vi "serialize.ob.cmd.vi"(11 "OrderBook.Commands.in":T1[](array[typedef])=[{"type"=enum."AddOrder", "side"=66, "orderId "=48, "quantity"=20000, "symbol"=4702127773838221344, "price"=9050, "executed.qty"=0, "canceled.qty"=0, "remaining.qty"=0, "seconds"=0, "nanoseconds"=0, "Add"=FALSE, "Edit"=FALSE, "Remove"=FALSE, "seq no"=0, "recv.time"=0, "parse.time"=0}] {"symbol" format="%.0x"; "orderId" format="%.0x"; "side" format="%.0x"}) -> (3 "Words.Out":u64[](array[numeric])=[1, 66, 48, 20000, 4702127773838221344, 9050, 0, 0, 0, 0, 0, 0, 0, 0, 0, 0, 2, 66, 48, 0, 0, 9050, 200, 0, 0, 0, 0, 0, 0, 0, 0, 0, 5, 66, 48, 1400, 6076284164848492576, 9050, 0, 0, 0, 0, 0, 0, 0, 0, 0, 0] format="%.0x")   [LabVIEW 2020, in "fpganow.common.host.lvlib"]
uses:
  fpganow.common.host.lvlib
  fpga/orderbook.command.ctl
  fpga/orderbook.command.type.ctl
  fpga/fpganow.common.fpga.lvlib
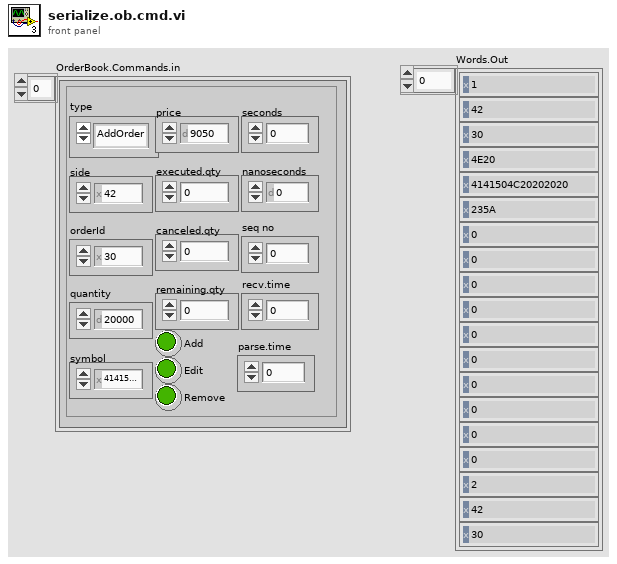
[diagram p1: front panel]
types:
  T1 = typedef "fpganow.common.fpga.lvlib/orderbook.command.ctl" = cluster{"type":T2, "side":u8, "orderId ":u64, "quantity":u32, "symbol":u64, "price":u64, "executed.qty":u32, "canceled.qty":u32, "remaining.qty":u32, "seconds":u64, "nanoseconds":u64, "Add":bool, "Edit":bool, "Remove":bool, "seq no":u32, "recv.time":u64, "parse.time":u64}
  T2 = typedef "fpganow.common.fpga.lvlib/orderbook.command.type.ctl" = enum8{"Time", "AddOrder", "OrderExecuted", "OrderExecutedAtPrice", "ReduceSize", "ModifyOrder", "DeleteOrder", "Get.Everything", "Get.All.Orders", "Get.Top"}
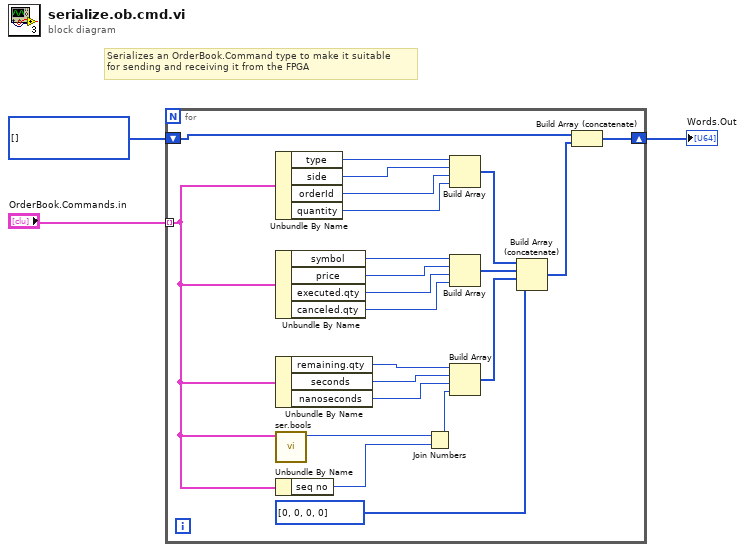
[diagram p0: block diagram]
diagram:
  # "Serializes an OrderBook.Command type to make it suitable\nfor sending and receiving it from the FPGA"
  n1 = for {
    tunnel: "OrderBook.Commands.in" -> [w6] mode=indexing
    shift-right: [w14] -> w1
    shift-left: u64[] [] -> [w16]
    n2 = Unbundle By Name(w6) -> ("type"=w12:T2, "side"=w11:u8, "orderId"=w10:u64, "quantity"=w9:u32)
    n3 = Unbundle By Name(w6) -> ("symbol"=w25:u64, "price"=w24:u64, "executed.qty"=w23:u32, "canceled.qty"=w22:u32)
    n4 = Unbundle By Name(w6) -> ("remaining.qty"=w21:u32, "seconds"=w20:u64, "nanoseconds"=w13:u64)
    n5 = call "ser.bools.vi"("orderbook.command"=w6) -> ("Numeric"=w7:u32)  [unwired: 10 in]
    n6 = Unbundle By Name(w6) -> ("seq no"=w5:u32)
    n7 = Join Numbers(hi=w7, lo=w5) -> ((hi.lo)=w8:u64)
    n8 = Build Array(w12, w11, w10, w9) -> (w19:u64[])
    n9 = Build Array(w25, w24, w23, w22) -> (w18:u64[])
    n10 = Build Array(w21, w20, w13, w8) -> (w17:u64[])
    n11 = Build Array (concatenate)(w19, w18, w17, u64[] [0, 0, 0, 0] ("array")) -> (w15:u64[])
    n12 = Build Array (concatenate)(w16, w15) -> (w14:u64[])
  }
  "Words.Out" <- w1
